vi "incident_conversion.vi"(9 "Offset":dbl, 11 "Voltage":string) -> (3 "Optical Power":string)   [LabVIEW 2017]
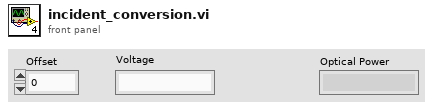
[diagram p1: front panel]
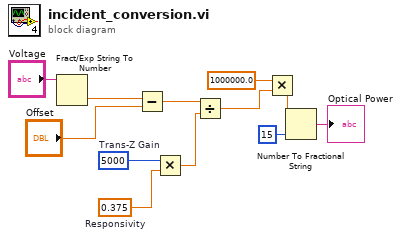
[diagram p0: block diagram]
diagram:
  w10 = 0.375  # Responsivity
  w11 = 5000  # Trans-Z Gain
  n1 = Fract/Exp String To Number(string="Voltage") -> (number=w3:dbl)  [unwired: 3 in, 1 out]
  n2 = Subtract(x=w3, y="Offset") -> (x-y=w4:dbl)
  n3 = Multiply(x=w11, y=w10) -> (x*y=w9:dbl)
  n4 = Divide(x=w4, y=w9) -> (x/y=w1:dbl)
  n5 = Multiply(x=1000000.0, y=w1) -> (x*y=w6:dbl)
  n6 = Number To Fractional String(number=w6, precision (6)=i16 15) -> (F-format string=→"Optical Power":string)  [unwired: 2 in]
